vi "ExampleInstrument.AppLauncher.vi"() -> ()   [LabVIEW 2016, in "ExampleInstrument.lvclass"]
uses:
  ExampleInstrument.lvclass
  <vilib>/JKI/JKI SMO/SMO/Typedefs/SMOState --Enum.ctl
  C:/Program Files (x86)/National Instruments/LabVIEW 2016/vi.lib/JKI/JKI SMO/SMO/SMO.lvclass
  C:/user/patrick/hg/levylab_inst/lvsrc/SMOs/Instrument/Instrument.lvclass
  Example Instrument UI/ExampleInstrument UI.lvclass
  C:/user/patrick/hg/levylab_inst/lvsrc/SMOs/Instrument UI/Instrument UI.lvclass
  C:/Program Files (x86)/National Instruments/LabVIEW 2016/vi.lib/JKI/JKI SMO/SMO.UI/SMO.UI.lvclass
  <vilib>/JKI/JKI SMO/SMO/SMO.lvclass
  <vilib>/JKI/JKI SMO/SMO.UI/SMO.UI.lvclass
  SMOs/Instrument UI/Instrument UI.lvclass
panel:
  out "error out":errorcluster
  in  "Splash Status":string="Push Start to Start..." caption="String"
  in  "Start":bool=TRUE
  in  "Stop":bool=TRUE
  out "UI SMO State":T1=enum."Stopped"
  out "SMO State":T1
  # "Example Instrument SMO Test Launcher"
  # "For instructions on how to use the JKI State Machine Objects, examples and video tutorials, visit:\nhttp://jki.net/state-machine-objects/\n\nJKI State Machine Objects™\nhttp://jki.net/state-machine-objects/\nCopyright (C) 2005-2015, JKI <info@jki.net>\nALL RIGHTS RESERVED"
  # "Starting Example Instrument..."
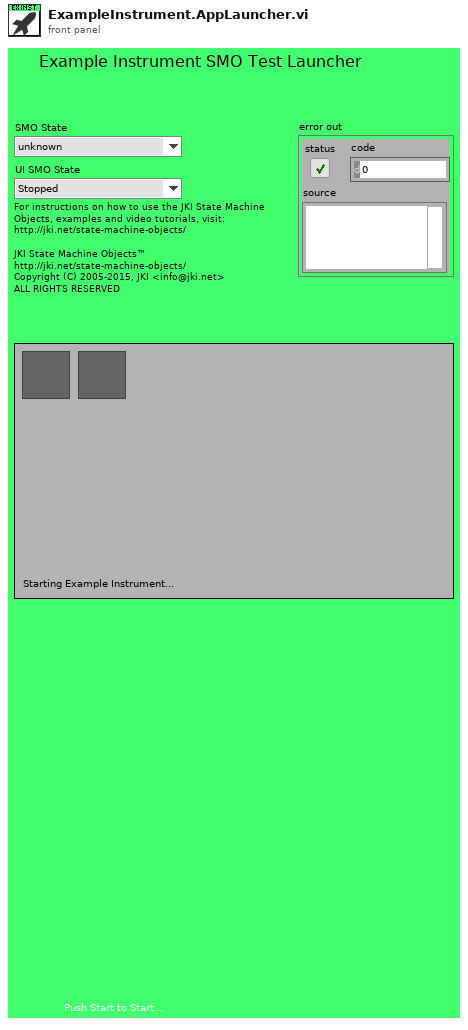
[diagram p1: front panel]
types:
  T1 = typedef "SMO.lvclass/SMOState --Enum.ctl" = enum16{"unknown", "Created", "Started", "Stopped"}
  T2 = enum32{"Invalid", "Standard", "Closed", "Hidden", "Minimized", "Maximized"}
  T3 = enum32{"invalid app kind", "Development System", "Run Time System", "Student Edition", "Embedded LabVIEW", "Evaluation", "Custom"}
  T4 = cluster{"Core":cluster{"Current VI Reference":refnum<vi>, "Close Panel on Exit?":bool}, "Instrument":refnum<class "ExampleInstrument.lvclass">, "Instrument UI":refnum<class "ExampleInstrument UI.lvclass">}
  T5 = cluster{"Current VI Reference":refnum<vi>, "Close Panel on Exit?":bool}
  T6 = typedef "SMO.lvclass/Public Events.ctl" = cluster{"Error":refnum<user-event>, "State":refnum<user-event>, "Reserve State":refnum<user-event>}
  T7 = cluster{"Event Registration Refnum":refnum<event-registration>, "Event Registration Refnum":refnum<event-registration>}
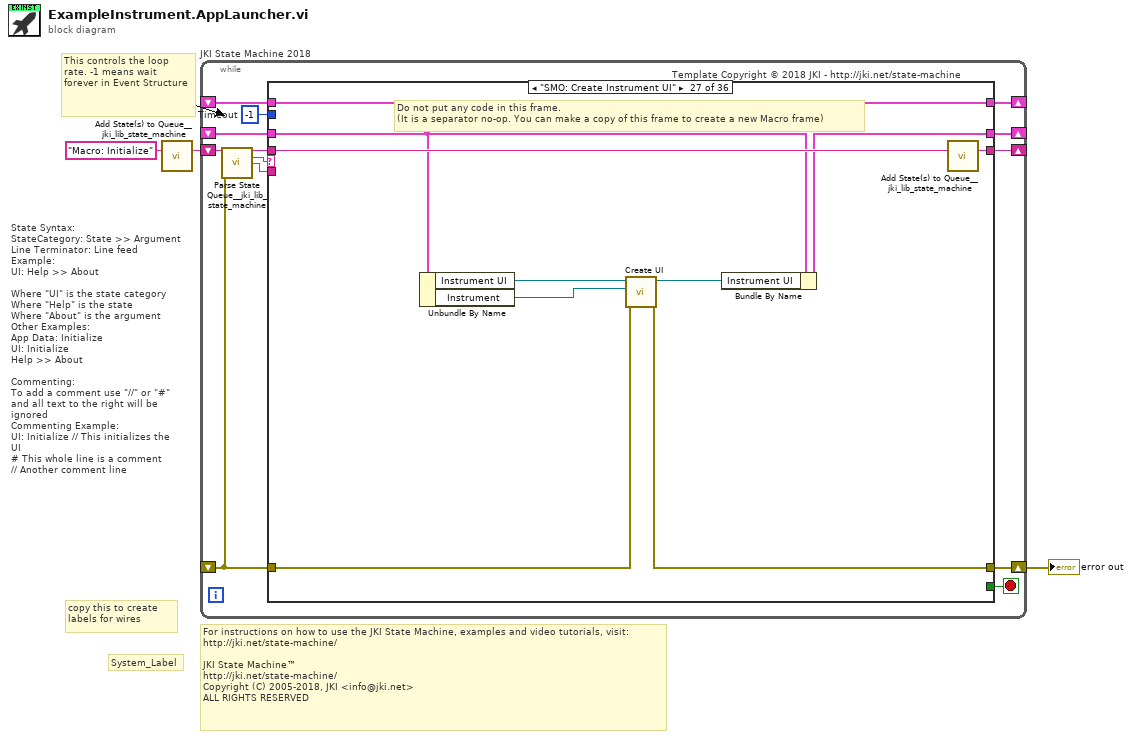
[diagram p0: block diagram]
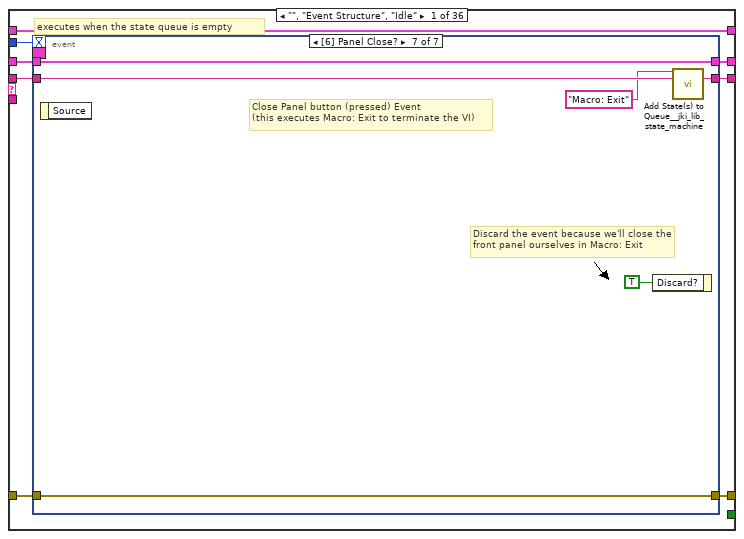
[diagram p2: hidden frame]
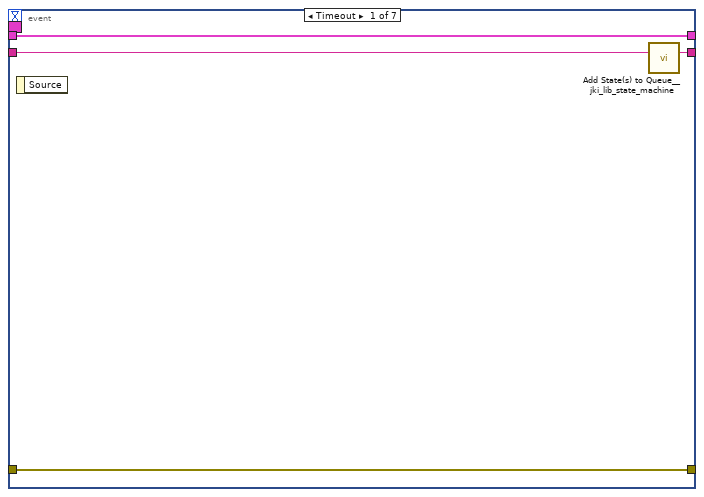
[diagram p3: hidden frame]
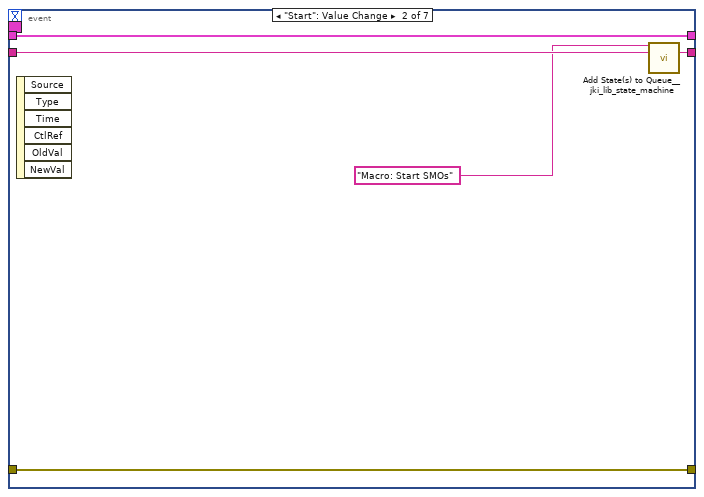
[diagram p4: hidden frame]
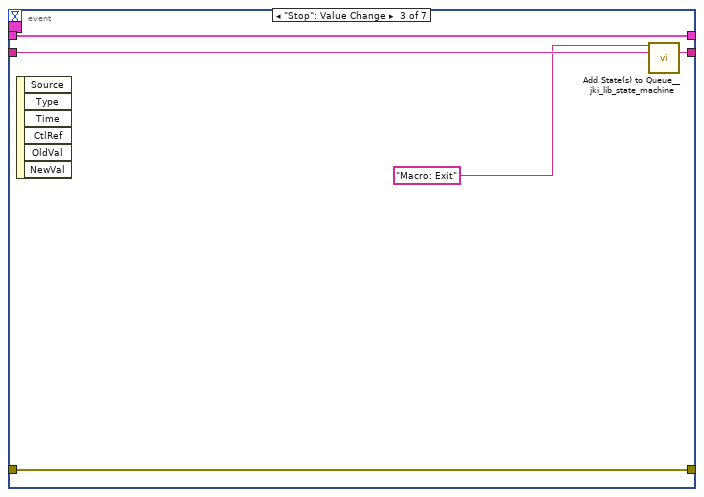
[diagram p5: hidden frame]
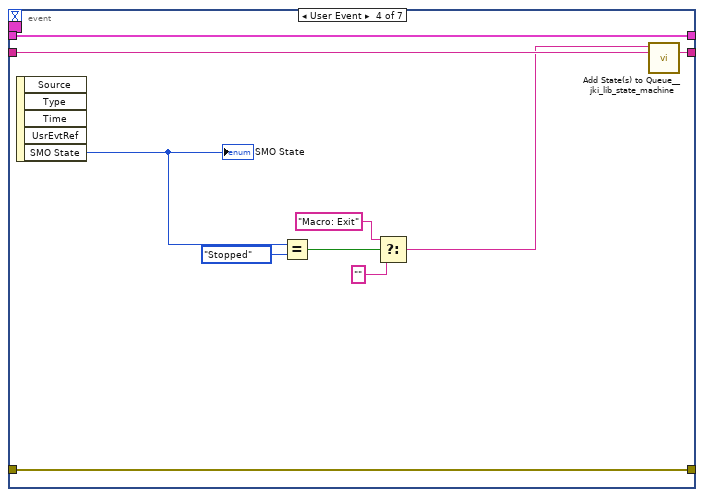
[diagram p6: hidden frame]
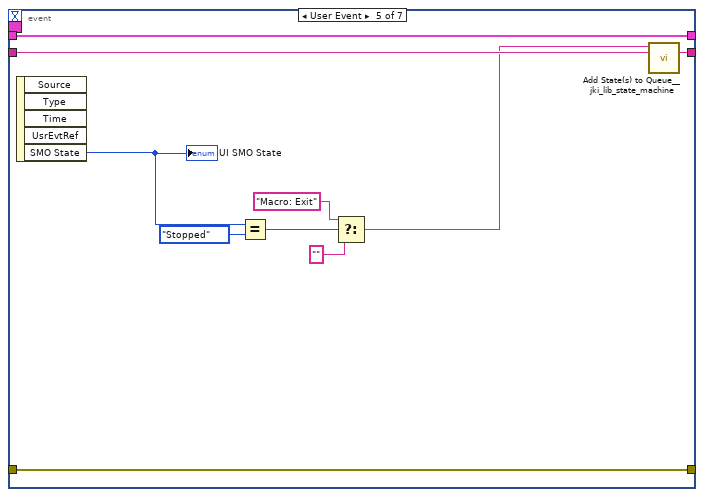
[diagram p7: hidden frame]
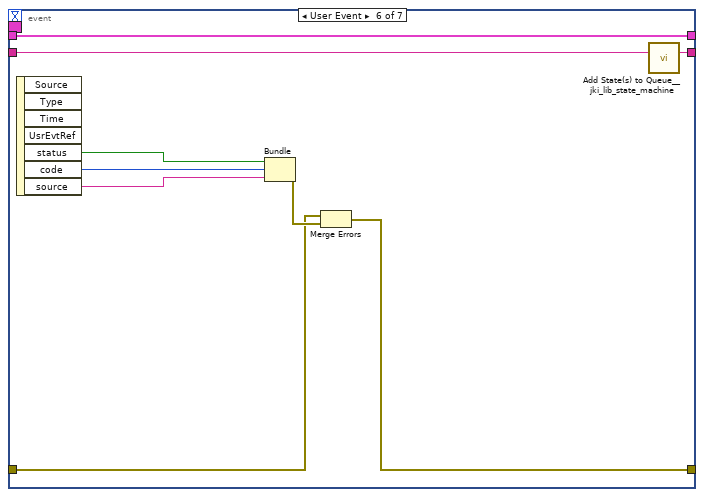
[diagram p8: hidden frame]
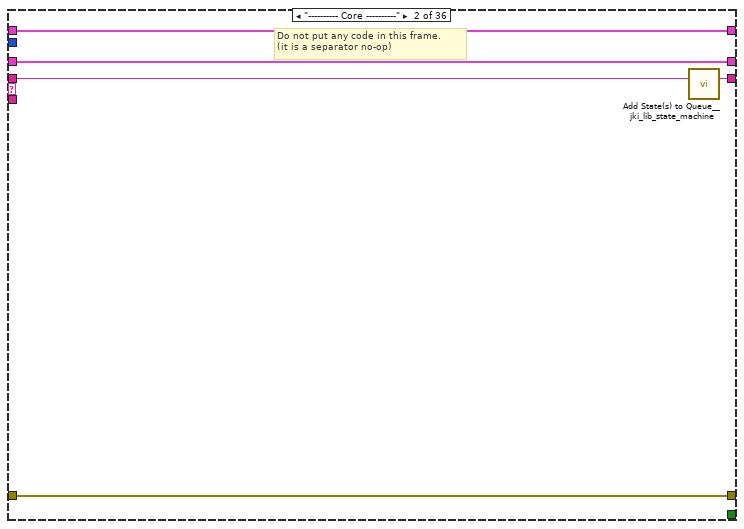
[diagram p9: hidden frame]
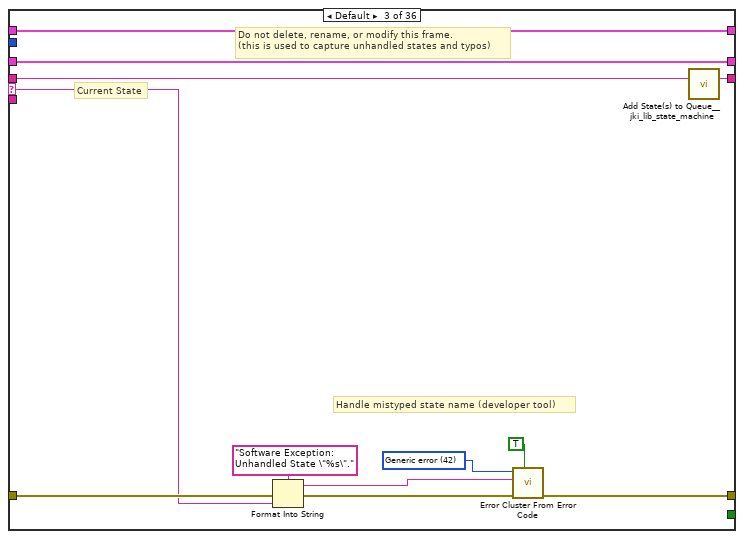
[diagram p10: hidden frame]
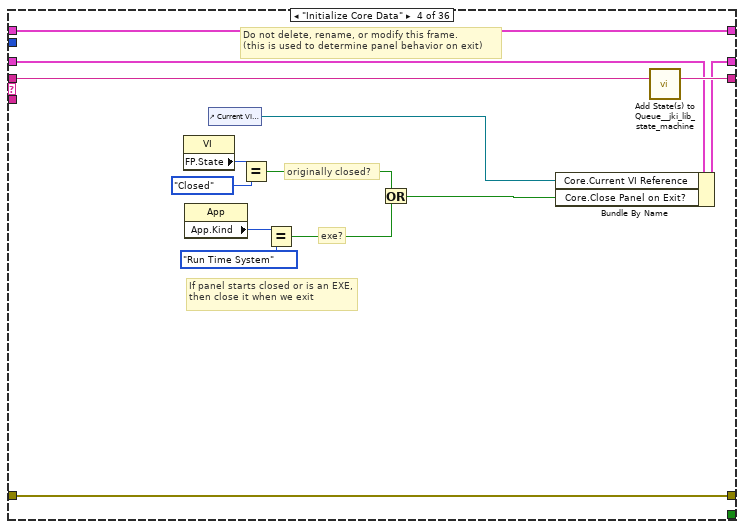
[diagram p11: hidden frame]
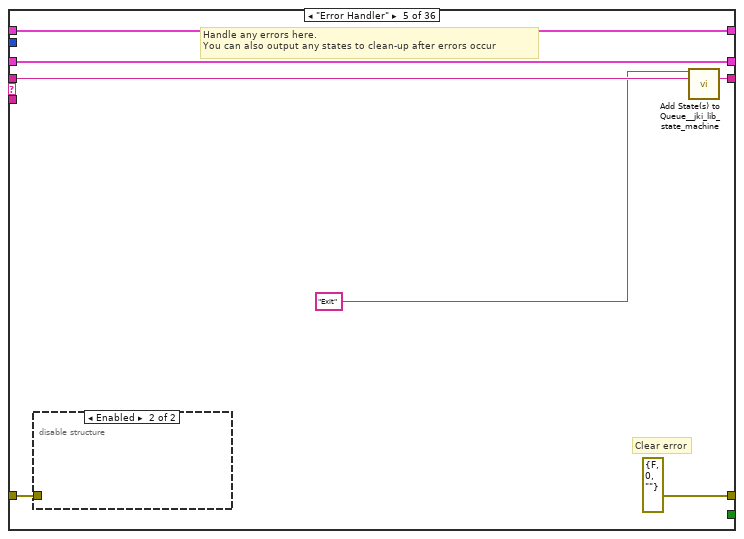
[diagram p12: hidden frame]
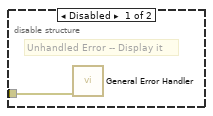
[diagram p13: hidden frame]
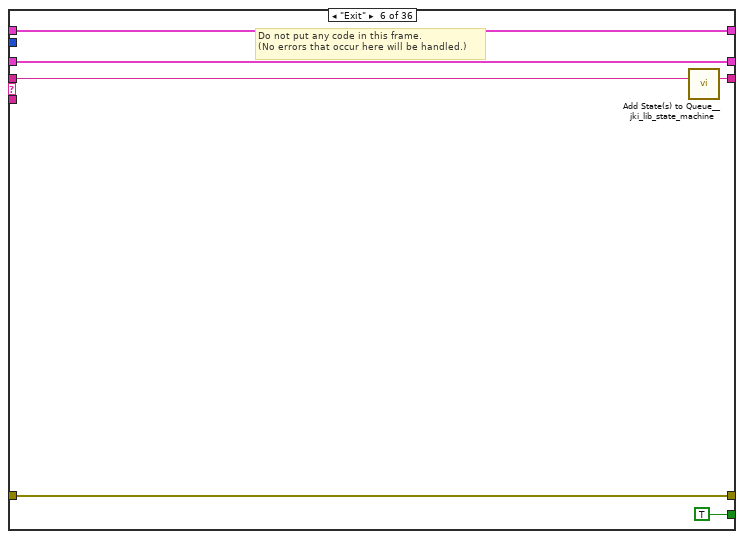
[diagram p14: hidden frame]
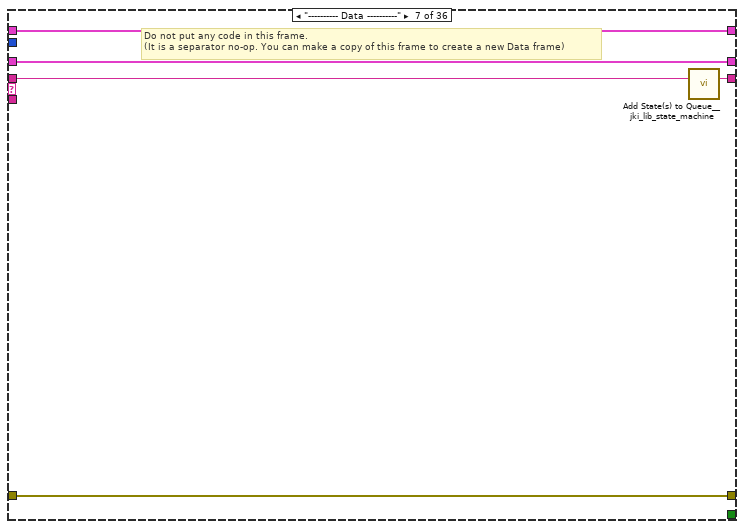
[diagram p15: hidden frame]
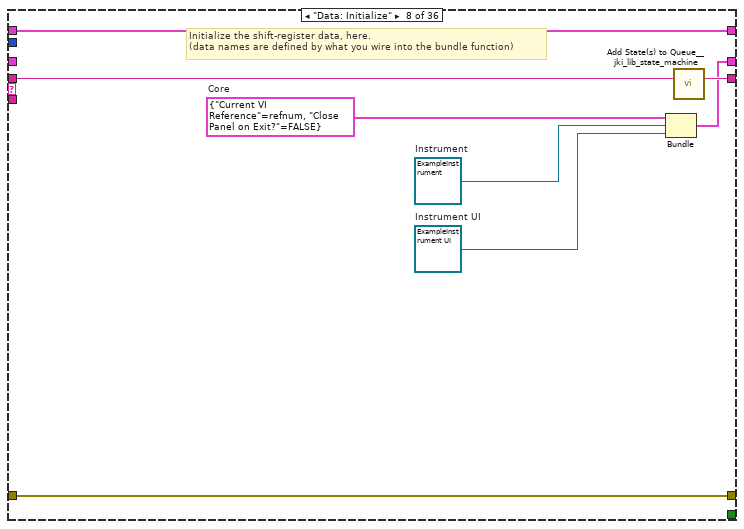
[diagram p16: hidden frame]
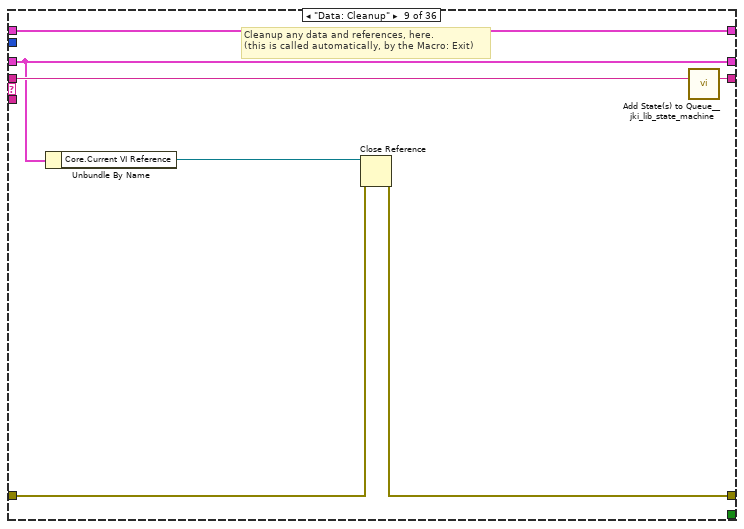
[diagram p17: hidden frame]
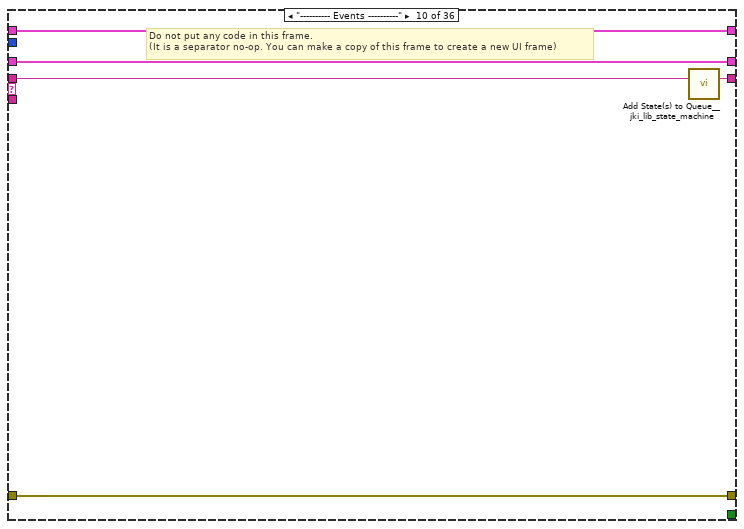
[diagram p18: hidden frame]
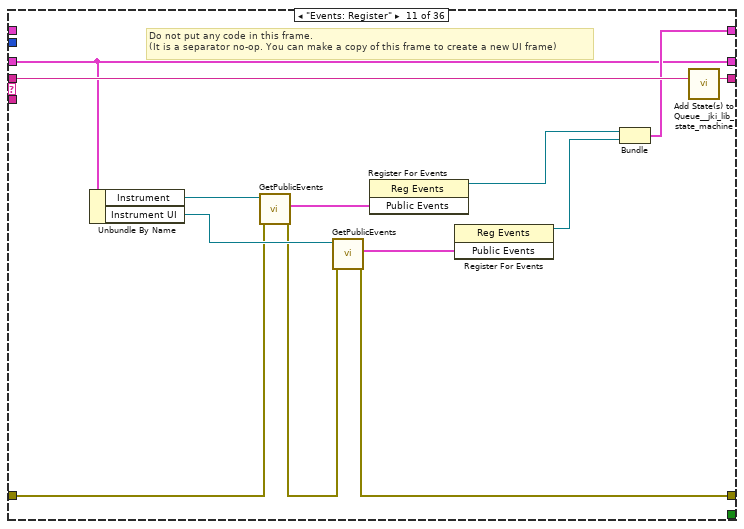
[diagram p19: hidden frame]
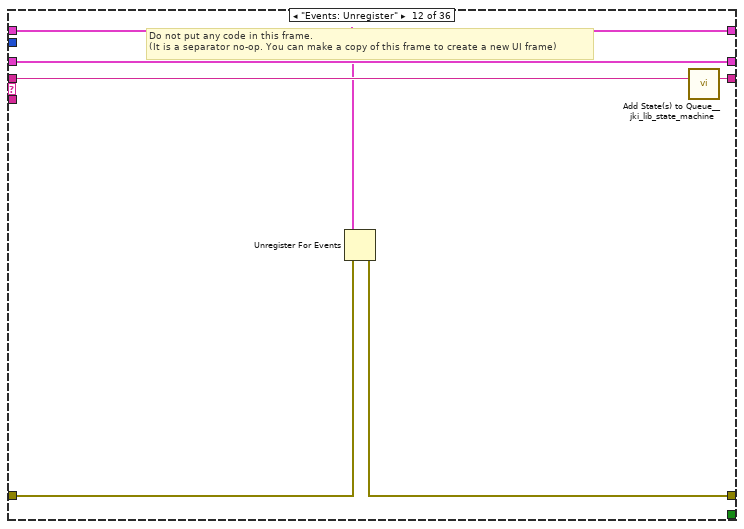
[diagram p20: hidden frame]
diagram:
  # "For instructions on how to use the JKI State Machine, examples and video tutorials, visit:\nhttp://jki.net/state-machine/\n\nJKI State Machine™\nhttp://jki.net/state-machine/\nCopyright (C) 2005-2018, JKI <info@jki.net>\nALL RIGHTS RESERVED"
  # "State Syntax:\nStateCategory: State >> Argument\nLine Terminator: Line feed\nExample:\nUI: Help >> About\n\nWhere \"UI\" is the state category\nWhere \"Help\" is the state\nWhere \"About\" is the argument\nOther Examples:\nApp Data: Initialize\nUI: Initialize\nHelp >> About\n\nCommenting:\nTo add a comment use \"//\" or \"#\" and all text to the right will be ignored\nCommenting Example:\nUI: Initialize // This initializes the UI\n# This whole line is a comment\n// Another comment line"
  # "copy this to create labels for wires"
  # "This controls the loop rate. -1 means wait forever in Event Structure"
  # "System_Label"
  n1 = call <vilib>:"Add State(s) to Queue__jki_lib_state_machine.vi"("State(s) in (\"\")"="Macro: Initialize") -> ("States Out"=w3:string)  [unwired: 14 in]
  n2 = while "JKI State Machine 2018" {
    shift-right: [w9] -> _
    shift-left: _ -> [w4]
    shift-right: [w12] -> w1
    shift-left: _ -> [w7]
    shift-right: [w11] -> _
    shift-left: w3 -> [w13]
    shift-right: [w6] -> _
    shift-left: _ -> [w5]
    stop <- w10 stop-if-true
    w8 = -1  # Timeout
    # "Template Copyright © 2018 JKI - http://jki.net/state-machine"
    n3 = call <vilib>:"Parse State Queue__jki_lib_state_machine.vi"("State Queue"=w13, "Error In (no error)"=w7) -> ("Remaining States"=w15:string, "Current State"=w16:string, "Arguments"=w14:string)  [unwired: 11 in]
    n4 = case shown="\"SMO: Create Instrument UI\"" w16 {
      selector: w16 -> [_ _ w80 _ _ _ _ _ _ _ _ _ _ _ _ _ _ _ _ _ _ _ _ _ _ _ _ _ _ _ _ _ _ _ _ _]
      tunnel: w15 -> [w24 w78 w84 w104 w111 w118 w123 w131 w138 w143 w156 w162 w167 w173 w180 w192 w270 w275 w280 w286 w292 w298 w310 w315 w326 w335 w345 w352 w363 w378 w393 w408 w423 w432 w439 w444]
      tunnel: w14 -> [_ _ _ _ _ _ _ _ _ _ _ _ _ _ w175 w186 _ _ _ _ _ _ _ _ _ _ _ _ _ _ _ _ _ _ w436 _]
      tunnel: [w21 w76 w86 w101 errorcluster {"status"=FALSE, "code"=0, "source"=""} ("error out") w115 w121 w126 w134 w141 w145 w157 w165 w168 w176 w189 w260 w273 w278 w284 w290 w296 w308 w313 w322 w327 w336 w346 w359 w374 w389 w405 w420 w430 w434 w442] -> w12
      tunnel: w7 -> [w20 w76 w85 w101 w107 w115 w121 w126 w135 w141 w147 w158 w165 w170 w177 w190 w261 w273 w278 w284 w290 w296 w308 w313 w323 w328 w337 w347 w356 w370 w386 w403 w416 w430 w435 w442]
      tunnel: [w23 w77 w83 w103 w110 w117 w122 w130 w137 w142 w155 w161 w166 w172 w179 w191 w269 w274 w279 w285 w291 w297 w309 w314 w325 w334 w344 w351 w362 w377 w392 w407 w422 w431 w438 w443] -> w11
      tunnel: [_ _ _ _ _ TRUE _ _ _ _ _ _ _ _ _ _ _ _ _ _ _ _ _ _ _ _ _ _ _ _ _ _ _ _ _ _] -> w10
      tunnel: [w19 w75 w82 w102 w108 w116 w120 w129 w133 w140 w150 w160 w164 w171 w178 w188 w258 w272 w277 w283 w289 w295 w307 w312 w321 w330 w341 w349 w360 w375 w390 w404 w419 w429 w437 w441] -> w9
      tunnel: w8 -> [w18 _ _ _ _ _ _ _ _ _ _ _ _ _ _ _ _ _ _ _ _ _ _ _ _ _ _ _ _ _ _ _ _ _ _ _]
      tunnel: [w17 w74 w79 w91 w105 w113 w119 w127 w132 w139 w153 w159 w163 w169 w174 w185 w259 w271 w276 w281 w288 w294 w301 w311 w324 w333 w343 w350 w361 w376 w391 w406 w421 w428 w433 w440] -> w6
      tunnel: w5 -> [w17 w74 w79 w91 w105 w113 w119 w127 w132 w139 _ w159 w163 w169 w174 w185 w259 w271 w276 w281 w288 w294 w301 w311 w324 w333 w343 w350 w361 w376 w391 w406 w421 w428 w433 w440]
      tunnel: w4 -> [w22 w75 w82 w97 w108 w116 w120 _ w133 w140 w150 w160 w164 w171 w178 w188 w258 w272 w277 w283 w289 w295 w307 w312 w319 w331 w342 w349 w360 w375 w390 w404 w419 w429 w437 w441]
      frame "", "Event Structure", "Idle" {
        # "executes when the state queue is empty"
        n5 = event shown="[6] Panel Close?" {
          selector: w17 -> [_ _ _ _ _ _ _]
          dyn-events: _ -> [_ _ _ _ _ _ _]
          timeout: w18 -> [_ _ _ _ _ _ _]
          tunnel: w24 -> [w28 w33 w38 w48 w58 w67 w73]
          tunnel: [w27 w32 w37 w47 w57 w66 w72] -> w23
          tunnel: w22 -> [w25 w30 w35 w45 w55 w65 w70]
          tunnel: [w26 w31 w36 w46 w56 w62 w71] -> w21
          tunnel: w20 -> [w26 w31 w36 w46 w56 w63 w71]
          tunnel: [w25 w30 w35 w45 w55 w65 w70] -> w19
          event Timeout {
            n6 = event-data() -> ()  [unwired: 1 in, 1 out]
            n7 = call <vilib>:"Add State(s) to Queue__jki_lib_state_machine.vi"("State(s) in (\"\")"=w28) -> ("States Out"=w27:string)  [unwired: 14 in]
          }
          event "Start": Value Change {
            n8 = event-data() -> ()  [unwired: 1 in, 6 out]
            n9 = call <vilib>:"Add State(s) to Queue__jki_lib_state_machine.vi"("State(s) in Front (\"\")"="Macro: Start SMOs" ("State(s) in Front (\"\")"), "State(s) in (\"\")"=w33) -> ("States Out"=w32:string)  [unwired: 13 in]
          }
          event "Stop": Value Change {
            n10 = event-data() -> ()  [unwired: 1 in, 6 out]
            n11 = call <vilib>:"Add State(s) to Queue__jki_lib_state_machine.vi"("State(s) in Front (\"\")"="Macro: Exit" ("State(s) in Front (\"\")"), "State(s) in (\"\")"=w38) -> ("States Out"=w37:string)  [unwired: 13 in]
          }
          event User Event {
            n12 = event-data() -> ("SMO State"=w40:T1)  [unwired: 1 in, 4 out]
            "SMO State" <- w40
            n13 = Equal?(x=w40, y=SMOState_--Enum."Stopped") -> (x = y?=w43:bool)
            n14 = Select(t="Macro: Exit", s=w43, f="" ("State(s) in Front (\"\")")) -> (s? t:f=w39:string)
            n15 = call <vilib>:"Add State(s) to Queue__jki_lib_state_machine.vi"("State(s) in Front (\"\")"=w39, "State(s) in (\"\")"=w48) -> ("States Out"=w47:string)  [unwired: 13 in]
          }
          event User Event {
            n16 = event-data() -> ("SMO State"=w49:T1)  [unwired: 1 in, 4 out]
            "UI SMO State" <- w49
            n17 = Equal?(x=w49, y=SMOState_--Enum."Stopped") -> (x = y?=w53:bool)
            n18 = Select(t="Macro: Exit", s=w53, f="" ("State(s) in Front (\"\")")) -> (s? t:f=w51:string)
            n19 = call <vilib>:"Add State(s) to Queue__jki_lib_state_machine.vi"("State(s) in Front (\"\")"=w51, "State(s) in (\"\")"=w58) -> ("States Out"=w57:string)  [unwired: 13 in]
          }
          event User Event {
            n20 = event-data() -> ("status"=w59:bool, "code"=w61:i32, "source"=w60:string)  [unwired: 1 in, 4 out]
            n21 = Bundle("status"=w59, "code"=w61, "source"=w60) -> (w64:errorcluster)  [unwired: 1 in]
            n22 = Merge Errors(w63, w64) -> (w62:errorcluster)
            n23 = call <vilib>:"Add State(s) to Queue__jki_lib_state_machine.vi"("State(s) in (\"\")"=w67) -> ("States Out"=w66:string)  [unwired: 14 in]
          }
          event Panel Close? {
            # "Discard the event because we'll close the front panel ourselves in Macro: Exit"
            # "Close Panel button (pressed) Event\n(this executes Macro: Exit to terminate the VI)"
            n24 = event-data() -> ()  [unwired: 1 in, 1 out]
            n25 = event-data("Discard?"=TRUE) -> ()  [unwired: 1 in, 1 out]
            n26 = call <vilib>:"Add State(s) to Queue__jki_lib_state_machine.vi"("State(s) in Front (\"\")"="Macro: Exit", "State(s) in (\"\")"=w73) -> ("States Out"=w72:string)  [unwired: 13 in]
          }
        }
      }
      frame "---------- Core ----------" {
        # "Do not put any code in this frame.\n(it is a separator no-op)"
        n27 = call <vilib>:"Add State(s) to Queue__jki_lib_state_machine.vi"("State(s) in (\"\")"=w78) -> ("States Out"=w77:string)  [unwired: 14 in]
      }
      frame Default {
        w89 = 42 items=["No error", "Argument error", "Memory is full", "Out of zone", "End of file", "File already open", "Generic file I/O error", "File not found", "File permission error", "Disk is full", "Duplicate path", "Too many files open", "System feature not enabled", "Resource file not found", "Cannot add resource", "Resource not found", "Image not found", "Image memory error", "Pen does not exist", "Config type invalid", "Config token not found", "Config parse error", "Config memory error", "Bad external code format", "Bad external code offset", "External code not present", "Null window", "Destroy window error", "Null menu", "Print aborted", "Bad print record", "Print driver error", "Windows error during printing", "Memory error during printing", "Print dialog error", "Generic print error", "Invalid device refnum", "Device not found", "Device parameter error", "Device unit error", "Cannot open device", "Device call aborted", "Generic error", "Cancelled by user", "Object ID too low", "Object ID too high", "Object not in heap", "Unknown heap", "Unknown object (invalid DefProc)", "Unknown object (DefProc not in table)", "Message out of range", "Invalid (null) method", "Unknown message", "Manager call not supported", "Bad address", "Network operation in progress", "Network operation timed out", "Connection is busy", "Network attribute not supported", "Network error", "Address in use", "System out of memory", "Connection aborted", "Connection refused", "Not connected", "Already connected", "Connection closed", "Initialization error (interapplication manager)", "Bad occurrence", "Wait on unbound occurrence handler", "Occurrence queue overflow", "Datalog type conflict", "Unused", "Unrecognized type (interapplication manager)", "Memory corrupt", "Failed to make temporary DLL", "Old CIN version", "Drag socket not found", "Failed to load drop-object", "Failed to register OLE object", "Failed to release OLE object", "Format specifier type mismatch", "Unknown format specifier", "Too few format specifiers", "Too many format specifiers", "Scan failed", "Newer CIN version", "Error converting to variant", "Runtime menu error", "Password tampered", "Variant attribute not found", "Incompatible variant data type", "Event data is not available", "Event Store is not present", "Occurrence is not found", "Event Queue is not created", "Event info is not available", "Refnum passed is NULL", "Error retrieving Class GUID", "Error retrieving CoClass GUID", "Error retrieving TypeLib GUID.", "Bad built application magic bytes.", "Specific driver is different from the specific driver associated with the Logical Name.", "There is no session opened to the class driver.", "Max Error", "MAX - Error with config objects", "MAX - Error loading configuration", "MAX - Group not supported"]
        # "Current State"
        # "Do not delete, rename, or modify this frame.\n(this is used to capture unhandled states and typos)"
        # "Handle mistyped state name (developer tool)"
        n28 = Format Into String(format string="Software Exception: Unhandled State \"%s\"." ("message"), error in=w85, w80) -> (resulting string=w88:string, error out=w87:errorcluster)  [unwired: 1 in]
        n29 = call <vilib>:"Error Cluster From Error Code.vi"("show call chain? (False)"=TRUE, "error in (no error)"=w87, "error message (\"\")"=w88, "error code (0)"=w89) -> ("error out"=w86:errorcluster)  [unwired: 5 in]
        n30 = call <vilib>:"Add State(s) to Queue__jki_lib_state_machine.vi"("State(s) in (\"\")"=w84) -> ("States Out"=w83:string)  [unwired: 14 in]
      }
      frame "Initialize Core Data" {
        # "Do not delete, rename, or modify this frame.\n(this is used to determine panel behavior on exit)"
        # "originally closed?"
        # "exe?"
        # "If panel starts closed or is an EXE, then close it when we exit"
        n31 = property class="VI"() -> ("FP.State"=w94:T2)  [unwired: 2 in, 2 out]
        n32 = property class="App"() -> ("App.Kind"=w100:T3)  [unwired: 2 in, 2 out]
        n33 = control-ref of="Current VI Reference"() -> (w95:refnum<vi>)
        n34 = Equal?(x=w94, y=T2."Closed" ("Front Panel Window:State")) -> (x = y?=w92:bool)
        n35 = Equal?(x=w100, y=T3."Run Time System" ("Application:Kind")) -> (x = y?=w98:bool)
        n36 = Or(x=w92, y=w98) -> (x .or. y?=w96:bool)
        n37 = Bundle By Name(cluster=w97, "Core.Current VI Reference"=w95, "Core.Close Panel on Exit?"=w96) -> (w102:T4)
        n38 = call <vilib>:"Add State(s) to Queue__jki_lib_state_machine.vi"("State(s) in (\"\")"=w104) -> ("States Out"=w103:string)  [unwired: 14 in]
      }
      frame "Error Handler" {
        # "Handle any errors here.\nYou can also output any states to clean-up after errors occur"
        # "Clear error"
        n39 = disable-structure shown="Enabled" {
          disable-tunnel: w107 -> [w112 _]
          frame Disabled {
            # "Unhandled Error -- Display it"
            n40 = call <vilib>:"General Error Handler.vi"("error in (no error)"=w112) -> ()  [unwired: 10 in, 5 out]
          }
          frame Enabled {
          }
        }
        n41 = call <vilib>:"Add State(s) to Queue__jki_lib_state_machine.vi"("State(s) in Front (\"\")"="Exit", "State(s) in (\"\")"=w111) -> ("States Out"=w110:string)  [unwired: 13 in]
      }
      frame "Exit" {
        # "Do not put any code in this frame.\n(No errors that occur here will be handled.)"
        n42 = call <vilib>:"Add State(s) to Queue__jki_lib_state_machine.vi"("State(s) in (\"\")"=w118) -> ("States Out"=w117:string)  [unwired: 14 in]
      }
      frame "---------- Data ----------" {
        # "Do not put any code in this frame.\n(It is a separator no-op. You can make a copy of this frame to create a new Data frame)"
        n43 = call <vilib>:"Add State(s) to Queue__jki_lib_state_machine.vi"("State(s) in (\"\")"=w123) -> ("States Out"=w122:string)  [unwired: 14 in]
      }
      frame "Data: Initialize" {
        w125 = refnum<class "ExampleInstrument UI.lvclass"> refnum  # Instrument UI
        w124 = refnum<class "ExampleInstrument.lvclass"> refnum  # Instrument
        w128 = T5 {"Current VI Reference"=refnum, "Close Panel on Exit?"=FALSE}  # Core
        # "Initialize the shift-register data, here.\n(data names are defined by what you wire into the bundle function)"
        n44 = Bundle("Core"=w128, "Instrument"=w124, "Instrument UI"=w125) -> (w129:T4)  [unwired: 1 in]
        n45 = call <vilib>:"Add State(s) to Queue__jki_lib_state_machine.vi"("State(s) in (\"\")"=w131) -> ("States Out"=w130:string)  [unwired: 14 in]
      }
      frame "Data: Cleanup" {
        # "Cleanup any data and references, here.\n(this is called automatically, by the Macro: Exit)"
        n46 = Unbundle By Name(w133) -> ("Core.Current VI Reference"=w136:refnum<vi>)
        n47 = Close Reference(reference=w136, error in (no error)=w135) -> (error out=w134:errorcluster)
        n48 = call <vilib>:"Add State(s) to Queue__jki_lib_state_machine.vi"("State(s) in (\"\")"=w138) -> ("States Out"=w137:string)  [unwired: 14 in]
      }
      frame "---------- Events ----------" {
        # "Do not put any code in this frame.\n(It is a separator no-op. You can make a copy of this frame to create a new UI frame)"
        n49 = call <vilib>:"Add State(s) to Queue__jki_lib_state_machine.vi"("State(s) in (\"\")"=w143) -> ("States Out"=w142:string)  [unwired: 14 in]
      }
      frame "Events: Register" {
        # "Do not put any code in this frame.\n(It is a separator no-op. You can make a copy of this frame to create a new UI frame)"
        n50 = Unbundle By Name(w150) -> ("Instrument"=w149:refnum<class "ExampleInstrument.lvclass">, "Instrument UI"=w148:refnum<class "ExampleInstrument UI.lvclass">)
        n51 = call <vilib>:"GetPublicEvents.vi"("error in (no error)"=w147, "SMO"=w149) -> ("error out"=w146:errorcluster, "Public Events"=w151:T6)  [unwired: 7 in, 1 out]
        n52 = call <vilib>:"GetPublicEvents.vi"("error in (no error)"=w146, "SMO"=w148) -> ("error out"=w145:errorcluster, "Public Events"=w152:T6)  [unwired: 7 in, 1 out]
        n53 = register-events(w151) -> (reference out=w154:refnum<event-registration>)  [unwired: 2 in, 1 out]
        n54 = register-events(w152) -> (reference out=w144:refnum<event-registration>)  [unwired: 2 in, 1 out]
        n55 = Bundle("Event Registration Refnum"=w154, "Event Registration Refnum"=w144) -> (w153:T7)  [unwired: 1 in]
        n56 = call <vilib>:"Add State(s) to Queue__jki_lib_state_machine.vi"("State(s) in (\"\")"=w156) -> ("States Out"=w155:string)  [unwired: 14 in]
      }
      frame "Events: Unregister" {
        # "Do not put any code in this frame.\n(It is a separator no-op. You can make a copy of this frame to create a new UI frame)"
        n57 = Unregister For Events(event registration refnum=w159, error in=w158) -> (error out=w157:errorcluster)
        n58 = call <vilib>:"Add State(s) to Queue__jki_lib_state_machine.vi"("State(s) in (\"\")"=w162) -> ("States Out"=w161:string)  [unwired: 14 in]
      }
      frame "---------- UI ----------" {
        # "Do not put any code in this frame.\n(It is a separator no-op. You can make a copy of this frame to create a new UI frame)"
        n59 = call <vilib>:"Add State(s) to Queue__jki_lib_state_machine.vi"("State(s) in (\"\")"=w167) -> ("States Out"=w166:string)  [unwired: 14 in]
      }
      frame "UI: Initialize" {
        # "Initialize the User Interface, here.\n(this is called automatically, by the Macro: Init)"
        n60 = invoke on="Stop" class="Bool (strict)" method="Reinit To Default"() -> ()  [unwired: 3 in, 3 out]
        n61 = invoke on="error out" class="Clust (strict)" method="Reinit To Default"() -> ()  [unwired: 3 in, 3 out]
        n62 = invoke on="SMO State 2" class="Enum (strict)" method="Reinit To Default"() -> ()  [unwired: 3 in, 3 out]
        n63 = invoke on="Start" class="Bool (strict)" method="Reinit To Default"() -> ()  [unwired: 3 in, 3 out]
        n64 = call <userlib>:"Fit VI window to Largest Dec__ogtk.vi"("error in (no error)"=w170) -> ("error out"=w168:errorcluster)  [unwired: 5 in, 1 out]
        n65 = call <vilib>:"Add State(s) to Queue__jki_lib_state_machine.vi"("State(s) in (\"\")"=w173) -> ("States Out"=w172:string)  [unwired: 14 in]
      }
      frame "UI: Cursor Set" {
        # "Argument"
        # "Set and Unset Cursor Busy.\n(Usage: \"UI: Cursor Set >> Busy|Idle\")"
        n66 = case shown="\"Idle\", Default" w175 {
          tunnel: w177 -> [w182 w184]
          tunnel: [w181 w183] -> w176
          frame "Idle", Default {
            n67 = call <vilib>:"Unset Busy.vi"("error in (no error)"=w182) -> ("error out"=w181:errorcluster)  [unwired: 10 in]
          }
          frame "Busy" {
            n68 = call <vilib>:"Set Busy.vi"("error in (no error)"=w184) -> ("error out"=w183:errorcluster)  [unwired: 9 in, 1 out]
          }
        }
        n69 = call <vilib>:"Add State(s) to Queue__jki_lib_state_machine.vi"("State(s) in (\"\")"=w180) -> ("States Out"=w179:string)  [unwired: 14 in]
      }
      frame "UI: Front Panel State" {
        # "Argument"
        # "Set Front Panel Open or Closed\n(Usage: \"UI: Front Panel State >> Open|Close\")"
        n70 = Unbundle By Name(w188) -> ("Core.Current VI Reference"=w187:refnum<vi>)
        n71 = case shown="\"Maximize\", \"Maximized\"" w186 {
          tunnel: w190 -> [w198 w213 w224 w237 w250]
          tunnel: [w200 w214 w226 w239 w252] -> w189
          tunnel: w187 -> [w199 w211 w225 w238 w251]
          frame "Open", "Standard", Default {
            w193 = T2."Standard" ("State")
            n72 = property class="VI"(reference=w199, error in=w198) -> (reference out=w196:refnum<vi>, error out=w197:errorcluster, "FP.State"=w195:T2)
            n73 = Not Equal?(x=w195, y=w193) -> (x != y?=w194:bool)
            n74 = case shown="True" w194 {
              tunnel: [w204 w206] -> w200
              tunnel: w197 -> [w203 w206]
              tunnel: w196 -> [w202 _]
              tunnel: w193 -> [w201 _]
              frame True {
                n75 = invoke class="VI" method="FP.Open"(reference=w202, error in=w203, "Activate"=TRUE, "State"=w201) -> (error out=w204:errorcluster)  [unwired: 1 in, 4 out]
              }
              frame False {
              }
            }
          }
          frame "Close", "Closed" {
            n76 = property class="VI"(reference=w211, error in=w213) -> (reference out=w210:refnum<vi>, error out=w212:errorcluster, "FP.State"=w208:T2)
            n77 = Not Equal?(x=w208, y=T2."Closed" ("Front Panel Window:State")) -> (x != y?=w207:bool)
            n78 = case shown="True" w207 {
              tunnel: [w215 w218] -> w214
              tunnel: w212 -> [w215 w217]
              tunnel: w210 -> [_ w216]
              frame False {
              }
              frame True {
                n79 = invoke class="VI" method="FP.Close"(reference=w216, error in=w217) -> (error out=w218:errorcluster)  [unwired: 1 in, 2 out]
              }
            }
          }
          frame "Hidden", "Hide" {
            w219 = T2."Hidden" ("State")
            n80 = property class="VI"(reference=w225, error in=w224) -> (reference out=w222:refnum<vi>, error out=w223:errorcluster, "FP.State"=w221:T2)
            n81 = Not Equal?(x=w221, y=w219) -> (x != y?=w220:bool)
            n82 = case shown="True" w220 {
              tunnel: [w230 w231] -> w226
              tunnel: w223 -> [w229 w231]
              tunnel: w222 -> [w228 _]
              tunnel: w219 -> [w227 _]
              frame True {
                n83 = invoke class="VI" method="FP.Open"(reference=w228, error in=w229, "State"=w227) -> (error out=w230:errorcluster)  [unwired: 2 in, 4 out]
              }
              frame False {
              }
            }
          }
          frame "Minimize", "Minimized" {
            w232 = T2."Minimized" ("State")
            n84 = property class="VI"(reference=w238, error in=w237) -> (reference out=w235:refnum<vi>, error out=w236:errorcluster, "FP.State"=w234:T2)
            n85 = Not Equal?(x=w234, y=w232) -> (x != y?=w233:bool)
            n86 = case shown="True" w233 {
              tunnel: [w243 w244] -> w239
              tunnel: w236 -> [w242 w244]
              tunnel: w235 -> [w241 _]
              tunnel: w232 -> [w240 _]
              frame True {
                n87 = invoke class="VI" method="FP.Open"(reference=w241, error in=w242, "State"=w240) -> (error out=w243:errorcluster)  [unwired: 2 in, 4 out]
              }
              frame False {
              }
            }
          }
          frame "Maximize", "Maximized" {
            w245 = T2."Maximized" ("State")
            n88 = property class="VI"(reference=w251, error in=w250) -> (reference out=w248:refnum<vi>, error out=w249:errorcluster, "FP.State"=w247:T2)
            n89 = Not Equal?(x=w247, y=w245) -> (x != y?=w246:bool)
            n90 = case shown="True" w246 {
              tunnel: [w256 w257] -> w252
              tunnel: w249 -> [w255 w257]
              tunnel: w248 -> [w254 _]
              tunnel: w245 -> [w253 _]
              frame True {
                n91 = invoke class="VI" method="FP.Open"(reference=w254, error in=w255, "State"=w253) -> (error out=w256:errorcluster)  [unwired: 2 in, 4 out]
              }
              frame False {
              }
            }
          }
        }
        n92 = call <vilib>:"Add State(s) to Queue__jki_lib_state_machine.vi"("State(s) in (\"\")"=w192) -> ("States Out"=w191:string)  [unwired: 14 in]
      }
      frame "UI: Set Background Color" {
        # "Do not put any code in this frame.\n(It is a separator no-op. You can make a copy of this frame to create a new UI frame)"
        n93 = property class="VI"(error in=w261) -> (error out=w263:errorcluster, "Panel"=w264:refnum<vi>)  [unwired: 1 in, 1 out]
        n94 = property class="Pnl"(reference=w264, error in=w263) -> (error out=w262:errorcluster, "Panes[]"=w265:refnum<vi>[])  [unwired: 1 out]
        n95 = Index Array(array=w265, index=0) -> (element=w267:refnum<vi>)
        n96 = property class="Pane"(reference=w267, error in=w262, "PaneColor"=u32 16777238 ("Color Box")) -> (error out=w260:errorcluster)  [unwired: 1 out]
        n97 = call <vilib>:"Add State(s) to Queue__jki_lib_state_machine.vi"("State(s) in (\"\")"=w270) -> ("States Out"=w269:string)  [unwired: 14 in]
      }
      frame "UI: Exit" {
        # "Do not put any code in this frame.\n(It is a separator no-op. You can make a copy of this frame to create a new UI frame)"
        n98 = invoke on="Start" class="Bool (strict)" method="Reinit To Default"() -> ()  [unwired: 3 in, 3 out]
        n99 = invoke on="Stop" class="Bool (strict)" method="Reinit To Default"() -> ()  [unwired: 3 in, 3 out]
        n100 = call <vilib>:"Add State(s) to Queue__jki_lib_state_machine.vi"("State(s) in (\"\")"=w275) -> ("States Out"=w274:string)  [unwired: 14 in]
      }
      frame "---------- Macro ----------" {
        # "Do not put any code in this frame.\n(It is a separator no-op. You can make a copy of this frame to create a new Macro frame)"
        n101 = call <vilib>:"Add State(s) to Queue__jki_lib_state_machine.vi"("State(s) in (\"\")"=w280) -> ("States Out"=w279:string)  [unwired: 14 in]
      }
      frame "Macro: Initialize" {
        # "Initialization Macro\n(This is called once, when the VI starts)"
        n102 = call <vilib>:"Add State(s) to Queue__jki_lib_state_machine.vi"("State(s) in Front (\"\")"="Data: Initialize\nInitialize Core Data\n//Events: Register\nUI: Initialize\nUI: Front Panel State >> Open\nUI: Set Background Color\nSplash: Set Status >> Push Start to Start...", "State(s) in (\"\")"=w286) -> ("States Out"=w285:string)  [unwired: 13 in]
      }
      frame "Macro: Start SMOs" {
        # "Do not put any code in this frame.\n(It is a separator no-op. You can make a copy of this frame to create a new Macro frame)"
        n103 = call <vilib>:"Add State(s) to Queue__jki_lib_state_machine.vi"("State(s) in Front (\"\")"="Splash: Set Status >> Starting Instrument...\nSMO: Create Instrument\nSMO: Create Instrument UI\nEvents: Register\nSMO: Start Instrument\nSplash: Set Status >> Instrument Process Started...\nSplash: Set Status >> Starting User Interface...\nSMO: Start Instrument UI\nUI: Front Panel State >> Hide\nSMO: Show Instrument UI" ("State(s) in Front (\"\")"), "State(s) in (\"\")"=w292) -> ("States Out"=w291:string)  [unwired: 13 in]
      }
      frame "Macro: Stop SMOs" {
        # "Do not put any code in this frame.\n(It is a separator no-op. You can make a copy of this frame to create a new Macro frame)"
        n104 = call <vilib>:"Add State(s) to Queue__jki_lib_state_machine.vi"("State(s) in Front (\"\")"="SMO: Destroy Instrument\nSMO: Hide Instrument UI\nSMO: Stop Instrument UI\nSMO: Destroy Instrument UI" ("State(s) in Front (\"\")"), "State(s) in (\"\")"=w298) -> ("States Out"=w297:string)  [unwired: 13 in]
      }
      frame "Macro: Exit" {
        # "Exit Macro\n(This is called once, when the VI exits)"
        n105 = Unbundle By Name(w307) -> ("Core.Close Panel on Exit?"=w306:bool)
        n106 = Select(t="UI: Front Panel State >> Open", s=w306, f="") -> (s? t:f=w303:string)
        n107 = call <vilib>:"Add State(s) to Queue__jki_lib_state_machine.vi"("State(s) in Front (\"\")"="UI: Front Panel State >> Open\nUI: Exit", "State(s) in (\"\")"=w303, "State(s) at Back (\"\")"="Macro: Stop SMOs\nData: Cleanup\nEvents: Unregister\nExit") -> ("States Out"=w302:string)  [unwired: 12 in]
        n108 = call <vilib>:"Add State(s) to Queue__jki_lib_state_machine.vi"("State(s) in Front (\"\")"=w302, "State(s) in (\"\")"=w310) -> ("States Out"=w309:string)  [unwired: 13 in]
      }
      frame "---------- SMO ----------" {
        # "Do not put any code in this frame.\n(It is a separator no-op. You can make a copy of this frame to create a new Macro frame)"
        n109 = call <vilib>:"Add State(s) to Queue__jki_lib_state_machine.vi"("State(s) in (\"\")"=w315) -> ("States Out"=w314:string)  [unwired: 14 in]
      }
      frame "SMO: Create Instrument" {
        w316 = FALSE  # Debug Mode? [F]
        w317 = TRUE  # Configuration Window? [T]
        # "Do not put any code in this frame.\n(It is a separator no-op. You can make a copy of this frame to create a new Macro frame)"
        n110 = Unbundle By Name(w319) -> ("Instrument"=w318:refnum<class "ExampleInstrument.lvclass">)
        n111 = call-dynamic "Create Instrument.vi"("error in (no error)"=w323, "Debug Mode? [F]"=w316, "Configuration Window? [T]"=w317, "Instrument in"=w318) -> ("error out"=w322:errorcluster, "Instrument out"=w320:refnum<class "ExampleInstrument.lvclass">)  [unwired: 6 in]
        n112 = Bundle By Name(cluster=w319, "Instrument"=w320) -> (w321:T4)
        n113 = call <vilib>:"Add State(s) to Queue__jki_lib_state_machine.vi"("State(s) in (\"\")"=w326) -> ("States Out"=w325:string)  [unwired: 14 in]
      }
      frame "SMO: Start Instrument" {
        # "Do not put any code in this frame.\n(It is a separator no-op. You can make a copy of this frame to create a new Macro frame)"
        n114 = Unbundle By Name(w331) -> ("Instrument"=w332:refnum<class "ExampleInstrument.lvclass">)
        n115 = call <vilib>:"Start.vi"("error in (no error)"=w328, "SMO"=w332) -> ("error out"=w327:errorcluster, "SMO out"=w329:refnum<class "ExampleInstrument.lvclass">)  [unwired: 8 in]
        n116 = Bundle By Name(cluster=w331, "Instrument"=w329) -> (w330:T4)
        n117 = call <vilib>:"Add State(s) to Queue__jki_lib_state_machine.vi"("State(s) in (\"\")"=w335) -> ("States Out"=w334:string)  [unwired: 14 in]
      }
      frame "SMO: Create Instrument UI" {
        # "Do not put any code in this frame.\n(It is a separator no-op. You can make a copy of this frame to create a new Macro frame)"
        n118 = Unbundle By Name(w342) -> ("Instrument UI"=w340:refnum<class "ExampleInstrument UI.lvclass">, "Instrument"=w339:refnum<class "ExampleInstrument.lvclass">)
        n119 = call "Create UI.vi"("error in (no error)"=w337, "Instrument in"=w339, "Instrument UI"=w340) -> ("error out"=w336:errorcluster, "Instrument UI out"=w338:refnum<class "ExampleInstrument UI.lvclass">)  [unwired: 7 in]
        n120 = Bundle By Name(cluster=w342, "Instrument UI"=w338) -> (w341:T4)
        n121 = call <vilib>:"Add State(s) to Queue__jki_lib_state_machine.vi"("State(s) in (\"\")"=w345) -> ("States Out"=w344:string)  [unwired: 14 in]
      }
      frame "SMO: Start Instrument UI" {
        # "Do not put any code in this frame.\n(It is a separator no-op. You can make a copy of this frame to create a new Macro frame)"
        n122 = Unbundle By Name(w349) -> ("Instrument UI"=w348:refnum<class "ExampleInstrument UI.lvclass">)
        n123 = call <vilib>:"Start.vi"("error in (no error)"=w347, "SMO"=w348) -> ("error out"=w346:errorcluster)  [unwired: 8 in, 1 out]
        n124 = call <vilib>:"Add State(s) to Queue__jki_lib_state_machine.vi"("State(s) in (\"\")"=w352) -> ("States Out"=w351:string)  [unwired: 14 in]
      }
      frame "SMO: Show Instrument UI" {
        # "Do not put any code in this frame.\n(It is a separator no-op. You can make a copy of this frame to create a new Macro frame)"
        n125 = Unbundle By Name(w360) -> ("Instrument UI"=w358:refnum<class "ExampleInstrument UI.lvclass">)
        n126 = call <vilib>:"GetState.vi"("error in (no error)"=w356, "SMO"=w358) -> ("error out"=w354:errorcluster, "SMO State"=w353:T1, "SMO out"=w357:refnum<class "ExampleInstrument UI.lvclass">)  [unwired: 7 in]
        n127 = call <vilib>:"Clear Errors.vi"("error in (no error)"=w354) -> ("error out"=w355:errorcluster)  [unwired: 5 in, 1 out]
        n128 = case shown="Default" w353 {
          tunnel: [w364 w367] -> w359
          tunnel: w357 -> [_ w366]
          tunnel: w355 -> [w364 w365]
          frame Default {
          }
          frame "Started" {
            n129 = call <vilib>:"Show.vi"("error in (no error)"=w365, "SMO.UI"=w366) -> ("error out"=w367:errorcluster)  [unwired: 8 in, 1 out]
          }
        }
        n130 = call <vilib>:"Add State(s) to Queue__jki_lib_state_machine.vi"("State(s) in (\"\")"=w363) -> ("States Out"=w362:string)  [unwired: 14 in]
      }
      frame "SMO: Destroy Instrument" {
        # "Do not put any code in this frame.\n(It is a separator no-op. You can make a copy of this frame to create a new Macro frame)"
        n131 = Unbundle By Name(w375) -> ("Instrument"=w373:refnum<class "ExampleInstrument.lvclass">)
        n132 = call <vilib>:"GetState.vi"("error in (no error)"=w370, "SMO"=w373) -> ("error out"=w369:errorcluster, "SMO State"=w372:T1, "SMO out"=w368:refnum<class "ExampleInstrument.lvclass">)  [unwired: 7 in]
        n133 = call <vilib>:"Clear Errors.vi"("error in (no error)"=w369) -> ("error out"=w371:errorcluster)  [unwired: 5 in, 1 out]
        n134 = case shown="Default" w372 {
          tunnel: [w379 w382] -> w374
          tunnel: w371 -> [w379 w381]
          tunnel: w368 -> [_ w380]
          frame Default {
          }
          frame "Stopped" {
            n135 = call <vilib>:"Destroy.vi"("error in (no error)"=w381, "SMO"=w380) -> ("error out"=w382:errorcluster)  [unwired: 9 in]
          }
        }
        n136 = call <vilib>:"Add State(s) to Queue__jki_lib_state_machine.vi"("State(s) in (\"\")"=w378) -> ("States Out"=w377:string)  [unwired: 14 in]
      }
      frame "SMO: Hide Instrument UI" {
        # "Do not put any code in this frame.\n(It is a separator no-op. You can make a copy of this frame to create a new Macro frame)"
        n137 = Unbundle By Name(w390) -> ("Instrument UI"=w388:refnum<class "ExampleInstrument UI.lvclass">)
        n138 = call <vilib>:"GetState.vi"("error in (no error)"=w386, "SMO"=w388) -> ("error out"=w384:errorcluster, "SMO State"=w383:T1, "SMO out"=w387:refnum<class "ExampleInstrument UI.lvclass">)  [unwired: 7 in]
        n139 = call <vilib>:"Clear Errors.vi"("error in (no error)"=w384) -> ("error out"=w385:errorcluster)  [unwired: 5 in, 1 out]
        n140 = case shown="Default" w383 {
          tunnel: [w394 w397] -> w389
          tunnel: w387 -> [_ w396]
          tunnel: w385 -> [w394 w395]
          frame Default {
          }
          frame "Started" {
            n141 = call <vilib>:"Hide.vi"("error in (no error)"=w395, "SMO.UI"=w396) -> ("error out"=w397:errorcluster)  [unwired: 8 in, 1 out]
          }
        }
        n142 = call <vilib>:"Add State(s) to Queue__jki_lib_state_machine.vi"("State(s) in (\"\")"=w393) -> ("States Out"=w392:string)  [unwired: 14 in]
      }
      frame "SMO: Stop Instrument UI" {
        # "Do not put any code in this frame.\n(It is a separator no-op. You can make a copy of this frame to create a new Macro frame)"
        n143 = Unbundle By Name(w404) -> ("Instrument UI"=w399:refnum<class "ExampleInstrument UI.lvclass">)
        n144 = call <vilib>:"GetState.vi"("error in (no error)"=w403, "SMO"=w399) -> ("error out"=w402:errorcluster, "SMO State"=w400:T1, "SMO out"=w398:refnum<class "ExampleInstrument UI.lvclass">)  [unwired: 7 in]
        n145 = call <vilib>:"Clear Errors.vi"("error in (no error)"=w402) -> ("error out"=w401:errorcluster)  [unwired: 5 in, 1 out]
        n146 = case shown="\"Created\", \"Started\"" w400 {
          tunnel: [w409 w412] -> w405
          tunnel: w398 -> [_ w411]
          tunnel: w401 -> [w409 w410]
          frame Default {
          }
          frame "Created", "Started" {
            n147 = call <vilib>:"Stop.vi"("error in (no error)"=w410, "SMO"=w411) -> ("error out"=w412:errorcluster)  [unwired: 8 in, 1 out]
          }
        }
        n148 = call <vilib>:"Add State(s) to Queue__jki_lib_state_machine.vi"("State(s) in (\"\")"=w408) -> ("States Out"=w407:string)  [unwired: 14 in]
      }
      frame "SMO: Destroy Instrument UI" {
        # "Do not put any code in this frame.\n(It is a separator no-op. You can make a copy of this frame to create a new Macro frame)"
        n149 = Unbundle By Name(w419) -> ("Instrument UI"=w418:refnum<class "ExampleInstrument UI.lvclass">)
        n150 = call <vilib>:"GetState.vi"("error in (no error)"=w416, "SMO"=w418) -> ("error out"=w415:errorcluster, "SMO State"=w413:T1, "SMO out"=w417:refnum<class "ExampleInstrument UI.lvclass">)  [unwired: 7 in]
        n151 = call <vilib>:"Clear Errors.vi"("error in (no error)"=w415) -> ("error out"=w414:errorcluster)  [unwired: 5 in, 1 out]
        n152 = case shown="Default" w413 {
          tunnel: w414 -> [w424 w427]
          tunnel: [w424 w426] -> w420
          tunnel: w417 -> [_ w425]
          frame Default {
          }
          frame "Stopped" {
            n153 = call <vilib>:"Destroy.vi"("error in (no error)"=w427, "SMO"=w425) -> ("error out"=w426:errorcluster)  [unwired: 9 in]
          }
        }
        n154 = call <vilib>:"Add State(s) to Queue__jki_lib_state_machine.vi"("State(s) in (\"\")"=w423) -> ("States Out"=w422:string)  [unwired: 14 in]
      }
      frame "---------- Splash ----------" {
        # "Template Separator\n(You can make a copy of, or modify, this frame)"
        n155 = call <vilib>:"Add State(s) to Queue__jki_lib_state_machine.vi"("State(s) in (\"\")"=w432) -> ("States Out"=w431:string)  [unwired: 14 in]
      }
      frame "Splash: Set Status" {
        # "Your code here.\n(You can make a copy of, or modify, this frame)"
        n156 = property on="Splash Status" class="Str"(error in=w435, "Value"=w436) -> (error out=w434:errorcluster)  [unwired: 1 in, 1 out]
        n157 = call <vilib>:"Add State(s) to Queue__jki_lib_state_machine.vi"("State(s) in (\"\")"=w439) -> ("States Out"=w438:string)  [unwired: 14 in]
      }
      frame "Splash: 2" {
        # "Your code here.\n(You can make a copy of, or modify, this frame)"
        n158 = call <vilib>:"Add State(s) to Queue__jki_lib_state_machine.vi"("State(s) in (\"\")"=w444) -> ("States Out"=w443:string)  [unwired: 14 in]
      }
    }
  }
  "error out" <- w1
